vi "Generate log file path.vi"(8 "error in":errorcluster) -> (0 "error out":errorcluster, 3 "Log File Cluster":T1)   [LabVIEW 2016]
uses:
  Tests/Log File Cluster.ctl
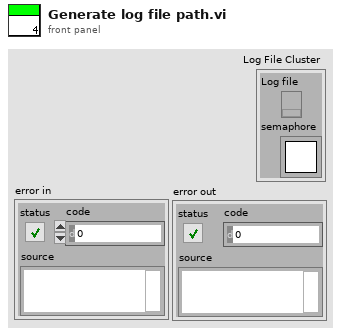
[diagram p1: front panel]
types:
  T1 = typedef "Log File Cluster.ctl" = cluster{"Log file":refnum<k34>, "semaphore":T2}
  T2 = typedef "Semaphore RefNum" = refnum<k1>
  T3 = enum16{"open", "open or create", "create or replace", "create", "open (read-only)"}
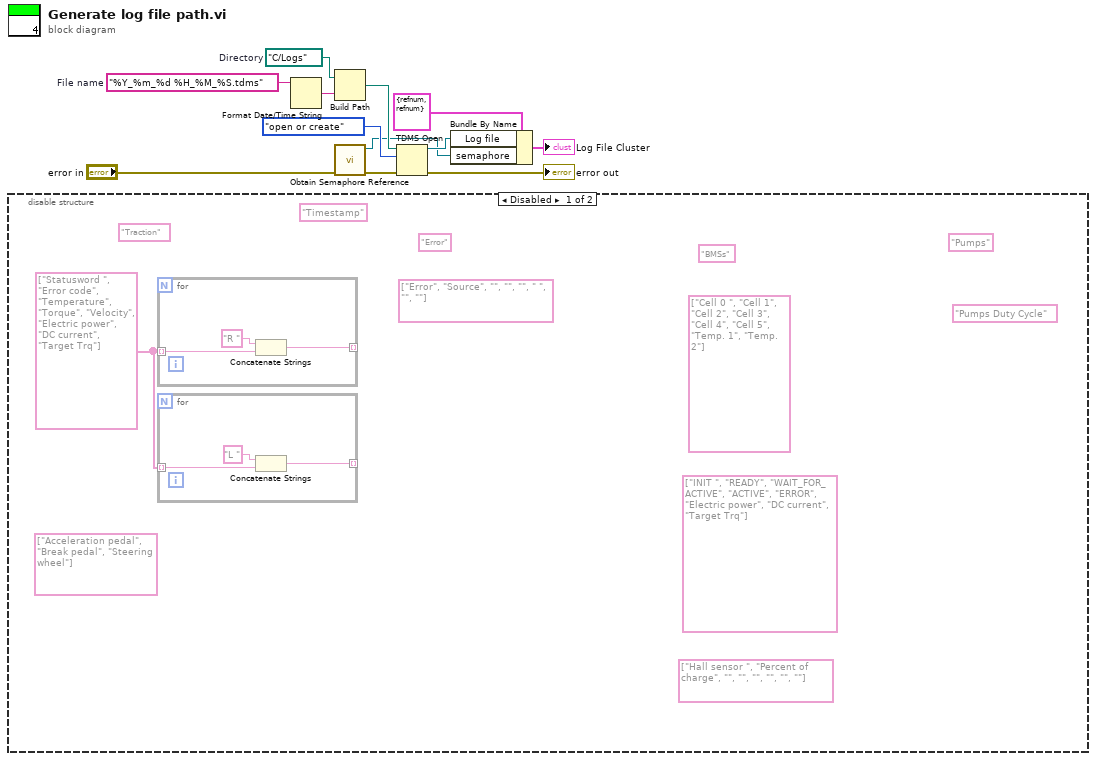
[diagram p0: block diagram]
diagram:
  w7 = path "C:/Logs"  # Directory
  w12 = "%Y_%m_%d %H_%M_%S.tdms"  # File name
  n1 = disable-structure shown="Disabled" {
    frame Disabled {
      (unwired) "Pumps"
      (unwired) "BMSs"
      (unwired) "Error"
      (unwired) "Traction"
      (unwired) "Pumps Duty Cycle"
      (unwired) string[] ["Error", "Source", "", "", "", " ", "", ""] ("channel name(s) in (Untitled)")
      (unwired) string[] ["Cell 0 ", "Cell 1", "Cell 2", "Cell 3", "Cell 4", "Cell 5", "Temp. 1", "Temp. 2"] ("channel name(s) in (Untitled)")
      (unwired) string[] ["Hall sensor ", "Percent of charge", "", "", "", "", "", ""] ("channel name(s) in (Untitled)")
      (unwired) string[] ["INIT ", "READY", "WAIT_FOR_ACTIVE", "ACTIVE", "ERROR", "Electric power", "DC current", "Target Trq"] ("channel name(s) in (Untitled)")
      (unwired) "Timestamp"
      (unwired) string[] ["Acceleration pedal", "Break pedal", "Steering wheel"]
      w13 = string[] ["Statusword ", "Error code", "Temperature", "Torque", "Velocity", "Electric power", "DC current", "Target Trq"] ("channel name(s) in (Untitled)")
      n2 = for {
        tunnel: w13 -> [w19] mode=indexing
        tunnel: [w17] -> _ mode=indexing
        n3 = Concatenate Strings("R " ("string"), w19) -> (w17:string)
      }
      n4 = for {
        tunnel: w13 -> [w16] mode=indexing
        tunnel: [w14] -> _ mode=indexing
        n5 = Concatenate Strings("L " ("string"), w16) -> (w14:string)
      }
    }
    frame Enabled {
    }
  }
  n6 = Format Date/Time String(time format string (%c)=w12) -> (date/time string=w11:string)  [unwired: 2 in]
  n7 = Build Path(base path=w7, name or relative path=w11) -> (appended path=w10:path)
  n8 = call <vilib>:"Obtain Semaphore Reference.vi"("error in (no error)"="error in") -> ("error out"=w5:errorcluster, "semaphore"=w1:T2)  [unwired: 4 in, 1 out]
  n9 = TDMS Open(8:w5, 10:T3."open or create" ("operation (0:open)"), 11:w10) -> (0:→"error out":errorcluster, 3:w2:refnum<k34>)  [unwired: 4 in]
  n10 = Bundle By Name(cluster=T1 {"Log file"=refnum, "semaphore"=refnum} ("Log File Cluster"), "Log file"=w2, "semaphore"=w1) -> (→"Log File Cluster":T1)
